vi "test Parse Sorted Object Dictionary_3.vi"(11 "Test Case In":refnum<class "test EDS.lvclass">) -> (0 "error out":errorcluster, 3 "Test Case Out":refnum<class "test EDS.lvclass">)   [LabVIEW 2024, in "test EDS.lvclass"]
uses:
  test EDS.lvclass
  C:/Program Files/National Instruments/LabVIEW 2024/vi.lib/Astemes/LUnit/Test Case.lvclass
  Core/EDS/EDS.lvclass
  Core/EDS/EDS.lvclass/EDS.ctl
  Core/Object Type.ctl
  <vilib>/Astemes/LUnit/Test Case.lvclass/Test Case.ctl
  <vilib>/Astemes/LUnit/Append Fail Result.vi
  <vilib>/Astemes/LUnit/Append Pass Result.vi
  <vilib>/Astemes/LUnit/Run In UI.vi
  <vilib>/Utility/error.llb/Clear Errors.vi
  Core/Sorted Object Dictionary/Sorted Object Dictionary.lvclass
  <vilib>/Astemes/LUnit/Test Case.lvclass
  Core/OD Entry/OD Entry.lvclass
  Core/EDS.lvlib
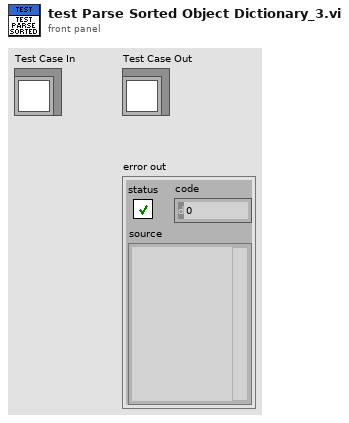
[diagram p1: front panel]
types:
  T1 = typedef "EDS.lvlib/Object Type.ctl" = u8
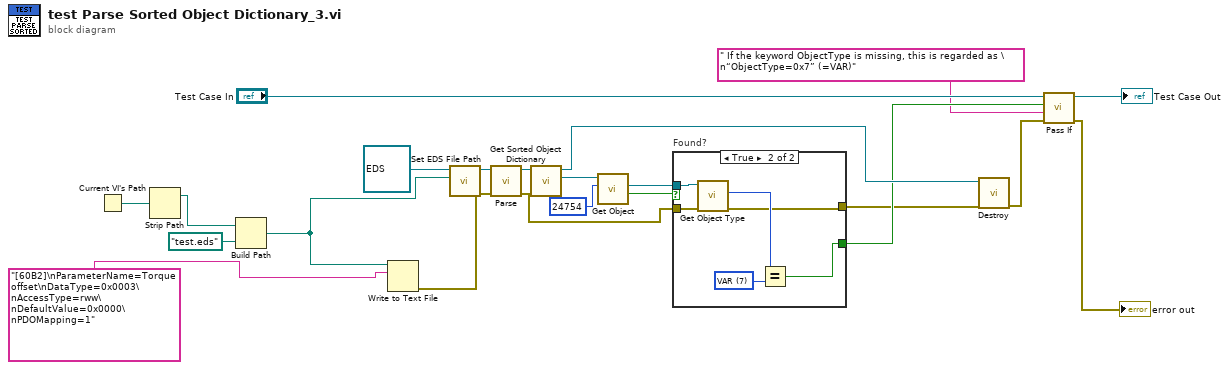
[diagram p0: block diagram]
diagram:
  n1 = Current VI's Path() -> (path=w17:path)
  n2 = Strip Path(path=w17) -> (stripped path=w13:path)  [unwired: 1 out]
  n3 = Build Path(base path=w13, name or relative path=path "test.eds") -> (appended path=w14:path)
  n4 = Write to Text File(file (use dialog)=w14, text="[60B2]\nParameterName=Torque offset\nDataType=0x0003\nAccessType=rww\nDefaultValue=0x0000\nPDOMapping=1") -> (error out=w15:errorcluster)  [unwired: 2 in, 2 out]
  n5 = call "Set EDS File Path.vi"("EDS File Path"=w14, "EDS in"=refnum<class "EDS.lvclass"> refnum ("EDS.lvlib:EDS.lvclass")) -> ("EDS out"=w18:refnum<class "EDS.lvclass">)  [unwired: 9 in]
  n6 = call "Parse.vi"("error in"=w15, "EDS in"=w18) -> ("error out"=w2:errorcluster, "EDS out"=w12:refnum<class "EDS.lvclass">)  [unwired: 8 in]
  n7 = call "Get Sorted Object Dictionary.vi"("EDS in"=w12) -> ("Sorted Object Dictionary"=w9:refnum<class "Sorted Object Dictionary.lvclass">, "EDS out"=w11:refnum<class "EDS.lvclass">)  [unwired: 9 in]
  n8 = call "Get Object.vi"("Numeric"=u16 24754, "Sorted Object Dictionary in"=w9) -> ("Found?"=w4:bool, "OD Entry"=w3:refnum<class "OD Entry.lvclass">)  [unwired: 7 in, 1 out]
  n9 = case "Found?" shown="True" w4 {
    selector: w4 -> [w23 _]
    tunnel: w3 -> [_ w30]
    tunnel: w2 -> [w24 w29]
    tunnel: [w23 w25] -> w7
    tunnel: [w24 w26] -> w5
    frame False {
    }
    frame True {
      w27 = T1 7 items=["NULL"=0, "DOMAIN"=2, "DEFTYPE"=5, "DEFSTRUCT"=6, "VAR"=7, "ARRAY"=8, "RECORD"=9] ("y")
      n10 = call "Get Object Type.vi"("Error In"=w29, "reference in"=w30) -> ("Error Out"=w26:errorcluster, "ObjectType"=w28:T1)  [unwired: 6 in, 2 out]
      n11 = Equal?(x=w28, y=w27) -> (x = y?=w25:bool)
    }
  }
  n12 = call "Destroy.vi"("error in"=w5, "EDS in"=w11) -> ("error out"=w6:errorcluster)  [unwired: 8 in, 1 out]
  n13 = call <vilib>:"Pass If.vi"("error in (no error)"=w6, "Message"=" If the keyword ObjectType is missing, this is regarded as \n“ObjectType=0x7” (=VAR)", "Pass?"=w7, "LUnit Test Case In"="Test Case In") -> ("error out"=→"error out":errorcluster, "LUnit Test Case Out"=→"Test Case Out":refnum<class "test EDS.lvclass">)  [unwired: 6 in]
